vi "LVSgettable.vi"(11 "Serial Port Select":refnum<visa-resource-name>="COM3") -> (0 "COM Error":bool, 2 "Sweep Table":dbl[][](array[numeric]) format="%#_6f")   [LabVIEW 2013]
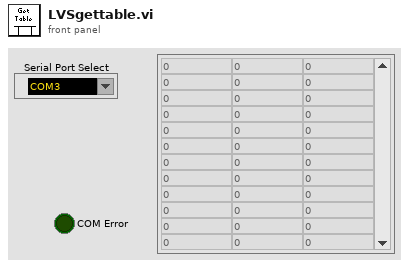
[diagram p1: front panel]
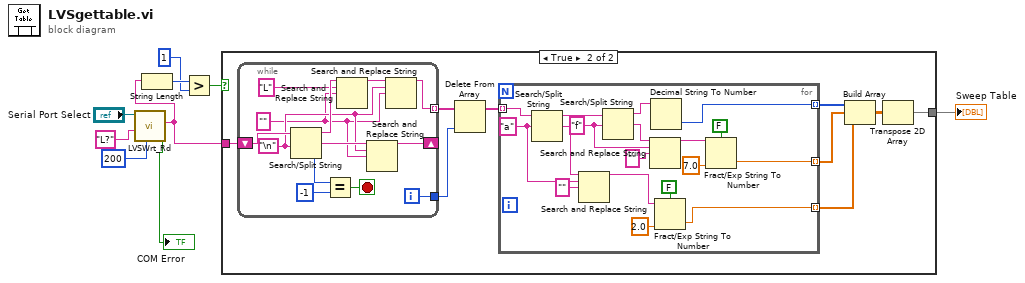
[diagram p0: block diagram]
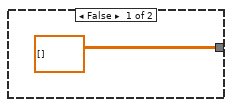
[diagram p2: hidden frame]
diagram:
  n1 = call "LVSWrt_Rd.vi"("delay"=u32 200, "WriteBuf"="L?" ("write buffer"), "COM Port"="Serial Port Select") -> ("ComError"=→"COM Error":bool, "string read"=w3:string)  [unwired: 7 in]
  n2 = String Length(string=w3) -> (length=w8:i32)
  n3 = Greater?(x=w8, y=1) -> (0:w9:bool)
  n4 = case shown="True" w9 {
    tunnel: w3 -> [_ w19]
    tunnel: [dbl[][] [] w11] -> w6
    frame False {
    }
    frame True {
      n5 = while {
        tunnel: [w44] -> w18 mode=indexing
        shift-right: [w41] -> _
        shift-left: w19 -> [w48]
        tunnel: [w38] -> w17
        i -> [w38]
        stop <- w50 stop-if-true
        w40 = "\n"
        w39 = "" ("replace string (\"\")")
        n6 = Search/Split String(string=w48, search string/char (-)=w40) -> (substring before match=w47:string, match + rest of string=w42:string, offset of match=w43:i32)  [unwired: 1 in]
        n7 = Equal?(x=w43, y=-1) -> (x = y?=w50:bool)
        n8 = Search and Replace String(input string=w47, search string="L" ("format string"), replace string=w39) -> (result string=w45:string)  [unwired: 5 in, 3 out]
        n9 = Search and Replace String(input string=w42, search string=w40, replace string=w39) -> (result string=w41:string)  [unwired: 5 in, 3 out]
        n10 = Search and Replace String(input string=w45, search string=w40, replace string=w39) -> (result string=w44:string)  [unwired: 5 in, 3 out]
      }
      n11 = Delete From Array(array=w18, index=w17) -> (array with subset deleted=w16:string[])  [unwired: 1 in, 1 out]
      n12 = for {
        tunnel: w16 -> [w37] mode=indexing
        tunnel: [w28] -> w15 mode=indexing
        tunnel: [w24] -> w14 mode=indexing
        tunnel: [w20] -> w13 mode=indexing
        w30 = "f" ("search string/char (-)")
        w34 = "a" ("search string/char (-)")
        n13 = Search/Split String(string=w37, search string/char (-)=w34) -> (substring before match=w36:string, match + rest of string=w35:string)  [unwired: 1 in, 1 out]
        n14 = Search and Replace String(input string=w35, search string=w34, replace string="" ("replace string (\"\")")) -> (result string=w21:string)  [unwired: 5 in, 3 out]
        n15 = Search/Split String(string=w36, search string/char (-)=w30) -> (substring before match=w29:string, match + rest of string=w31:string)  [unwired: 1 in, 1 out]
        n16 = Search and Replace String(input string=w31, search string=w30, replace string="" ("replace string (\"\")")) -> (result string=w25:string)  [unwired: 5 in, 3 out]
        n17 = Decimal String To Number(string=w29) -> (number=w28:i32)  [unwired: 2 in, 1 out]
        n18 = Fract/Exp String To Number(use system decimal point (T)=FALSE, string=w21, default (0 dbl)=2.0 ("default (0 DBL)")) -> (number=w20:dbl)  [unwired: 1 in, 1 out]
        n19 = Fract/Exp String To Number(use system decimal point (T)=FALSE, string=w25, default (0 dbl)=7.0 ("default (0 DBL)")) -> (number=w24:dbl)  [unwired: 1 in, 1 out]
      }
      n20 = Build Array(w15, w14, w13) -> (w12:dbl[][])
      n21 = Transpose 2D Array(2D array=w12) -> (transposed array=w11:dbl[][])
    }
  }
  "Sweep Table" <- w6
